vi "Experiment_2.vi"() -> ()   [LabVIEW 2019]
uses:
  <vilib>/measure/NI_MABase.lvlib
panel:
  out "Wave 3":waveform(dbl)(graph)={"t0"=timestamp(0 s since 1904-01-01), "dt"=0.001, "Y"=array[1000 elements]}
  out "Wave 2":waveform(dbl)(graph)={"t0"=timestamp(0 s since 1904-01-01), "dt"=0.001, "Y"=array[1000 elements]}
  out "Wave 1":waveform(dbl)(graph)={"t0"=timestamp(0 s since 1904-01-01), "dt"=0.001, "Y"=array[1000 elements]}
  out "Added Waves":waveform(dbl)(graph)={"t0"=timestamp(0 s since 1904-01-01), "dt"=0.001, "Y"=array[1000 elements]}
  in  "sampling info 3":cluster{"Fs":dbl, "#s":dbl}={"Fs"=1000.0, "#s"=1000.0} {"Fs" format="%.2p"}
  in  "sampling info 2":cluster{"Fs":dbl, "#s":dbl}={"Fs"=1000.0, "#s"=1000.0} {"Fs" format="%.2p"}
  in  "sampling info":cluster{"Fs":dbl, "#s":dbl}={"Fs"=1000.0, "#s"=1000.0} {"Fs" format="%.2p"}
  out "Retrieved Wave 3":dynamicdata(graph)=[{"t0"=timestamp(0 s since 1904-01-01), "dt"=0.001, "Y"=array[1000 elements], "attributes"=variant("NI_ChannelName"=variant(string "Filtered"))}]
  out "Retrieved Wave 2":dynamicdata(graph)=[{"t0"=timestamp(0 s since 1904-01-01), "dt"=0.001, "Y"=array[1000 elements], "attributes"=variant("NI_ChannelName"=variant(string "Filtered"))}]
  out "Retrieved Wave 1":dynamicdata(graph)=[{"t0"=timestamp(0 s since 1904-01-01), "dt"=0.001, "Y"=array[1000 elements], "attributes"=variant("NI_ChannelName"=variant(string "Filtered"))}]
  in  "signal type 3":T1(ring)
  in  "signal type 2":T1(ring)
  in  "signal type":T1(ring)
  in  "amplitude 4":dbl=1.0 format="%0.2p"
  in  "phase":dbl format="%.2p"
  in  "frequency":dbl=10.0 format="%0.2p"
  in  "phase 3":dbl format="%.2p"
  in  "amplitude 3":dbl=1.0 format="%0.2p"
  in  "frequency 3":dbl=100.0 format="%0.2p"
  in  "phase 2":dbl format="%.2p"
  in  "amplitude 2":dbl=1.0 format="%0.2p"
  in  "frequency 2":dbl=50.0 format="%0.2p"
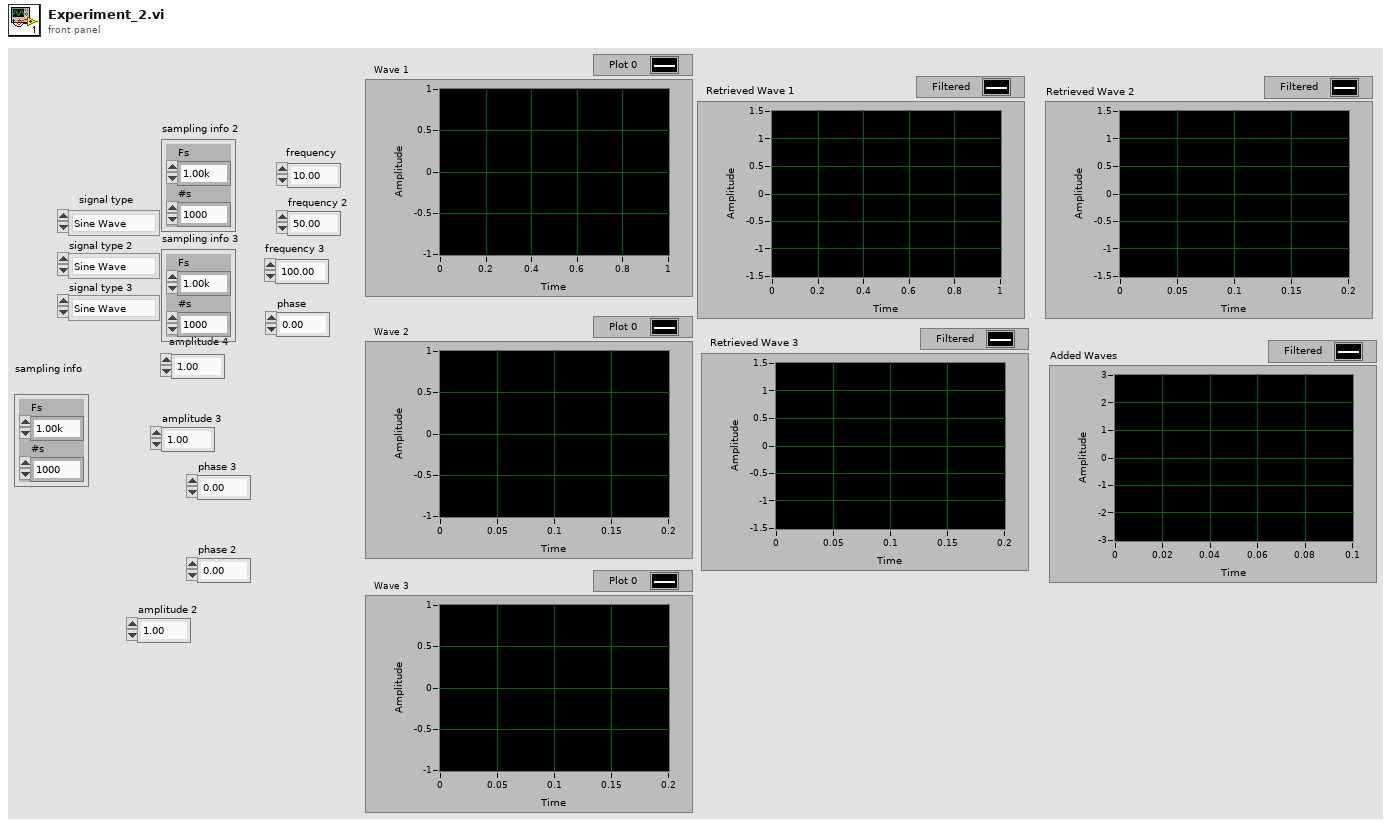
[diagram p1: front panel]
types:
  T1 = enum16{"Sine Wave", "Triangle Wave", "Square Wave", "Sawtooth Wave"}
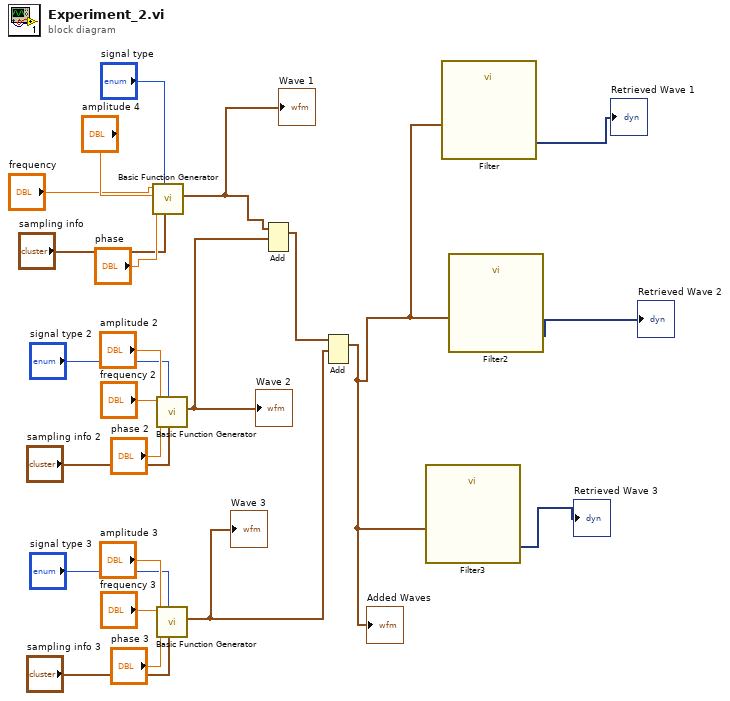
[diagram p0: block diagram]
diagram:
  n1 = call <vilib>:"Basic Function Generator.vi"("sampling info"="sampling info", "signal type"="signal type", "phase"="phase", "amplitude"="amplitude 4", "frequency"="frequency") -> ("signal out"=w1:waveform(dbl))  [unwired: 4 in, 2 out]
  "Wave 1" <- w1
  n2 = call <vilib>:"Basic Function Generator.vi"("sampling info"="sampling info 2", "signal type"="signal type 2", "phase"="phase 2", "amplitude"="amplitude 2", "frequency"="frequency 2") -> ("signal out"=w3:waveform(dbl))  [unwired: 4 in, 2 out]
  "Wave 2" <- w3
  n3 = call <vilib>:"Basic Function Generator.vi"("sampling info"="sampling info 3", "signal type"="signal type 3", "phase"="phase 3", "amplitude"="amplitude 3", "frequency"="frequency 3") -> ("signal out"=w2:waveform(dbl))  [unwired: 4 in, 2 out]
  "Wave 3" <- w2
  n4 = Add(1:w3, 2:w1) -> (0:w14:waveform(dbl))  [unwired: 1 in, 1 out]
  n5 = Add(1:w2, 2:w14) -> (0:w4:waveform(dbl))  [unwired: 1 in, 1 out]
  "Added Waves" <- w4
  n6 = call "Filter3"("Signal"=w4) -> ("Filtered Signal"=→"Retrieved Wave 3":dynamicdata)  [unwired: 9 in, 1 out]
  n7 = call "Filter"("Signal"=w4) -> ("Filtered Signal"=→"Retrieved Wave 1":dynamicdata)  [unwired: 9 in, 1 out]
  n8 = call "Filter2"("Signal"=w4) -> ("Filtered Signal"=→"Retrieved Wave 2":dynamicdata)  [unwired: 9 in, 1 out]
